vi "obtain_latest_instance.vi"(7 "quick, but maybe outdated?":bool=TRUE, 8 "error in (no error)":errorcluster) -> (0 "error out":errorcluster, 3 "GenericExperimentController out":refnum<class "GenericExperimentController.lvclass">)   [LabVIEW 2010, in "GenericExperimentController.lvclass"]
uses:
  GenericExperimentController.lvclass
  class_data.vi
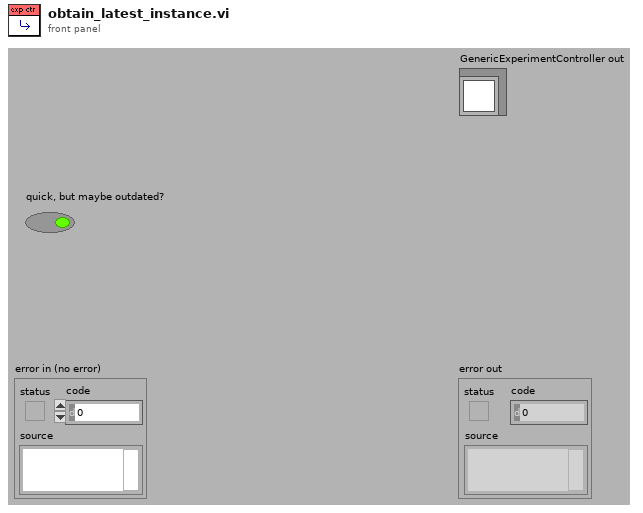
[diagram p1: front panel]
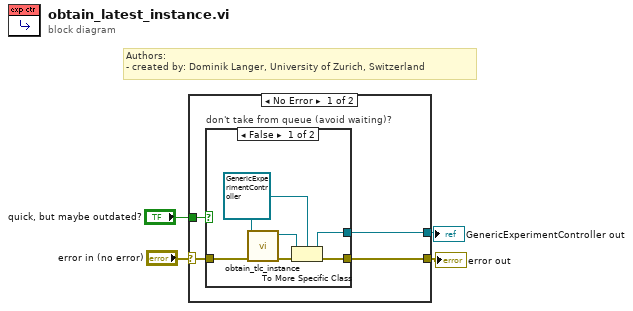
[diagram p0: block diagram]
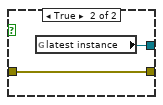
[diagram p2: hidden frame]
diagram:
  # "Authors:  \n- created by: Dominik Langer, University of Zurich, Switzerland"
  n1 = case shown="No Error" "error in (no error)" {
    selector: "error in (no error)" -> [w8 w17]
    tunnel: [w7 w17] -> w3
    tunnel: [w6 _] -> w2
    tunnel: "quick, but maybe outdated?" -> [w5 _]
    frame No Error {
      n2 = case "don't take from queue (avoid waiting)?" shown="False" w5 {
        tunnel: w8 -> [w10 w15]
        tunnel: [w12 w15] -> w7
        tunnel: [w11 w16] -> w6
        frame False {
          w9 = refnum<class "GenericExperimentController.lvclass"> refnum ("GenericExperimentController.lvclass")
          n3 = call-dynamic "obtain_tlc_instance.vi"("error in (no error)"=w10, "GenericToplevelComponent in"=w9) -> ("error out"=w14:errorcluster, "GenericToplevelComponent out"=w13:refnum<class "GenericToplevelComponent.lvclass">)  [unwired: 8 in]
          n4 = To More Specific Class(target class=w9, reference=w13, error in=w14) -> (specific class reference=w11:refnum<class "GenericExperimentController.lvclass">, error out=w12:errorcluster)
        }
        frame True {
          n5 = global read "class_data.vi" "latest instance"() -> (w16:refnum<class "GenericExperimentController.lvclass">)
        }
      }
    }
    frame Error {
    }
  }
  "error out" <- w3
  "GenericExperimentController out" <- w2
